vi "New JSON ([]).vi"(8 "error in (no error)":errorcluster) -> (0 "error out":errorcluster, 3 "JSON Value out":refnum<class "JSON Value.lvclass">)   [LabVIEW 2017, in "JSON Value.lvclass"]
doc: "Creates a new empty JSON Array"
uses:
  JSON Value.lvclass
  JSON Types.ctl
  JSON Value.lvclass/JSON Value.ctl
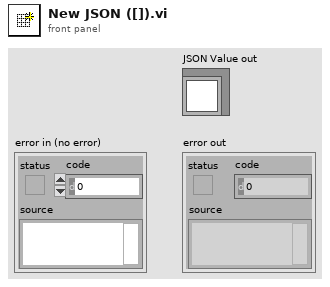
[diagram p1: front panel]
types:
  T1 = typedef "JSON Value.lvclass/JSON Types.ctl" = enum16{"String", "Numeric", "Boolean", "NULL", "Object", "Array"}
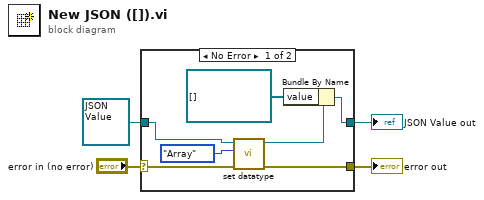
[diagram p0: block diagram]
diagram:
  n1 = case shown="No Error" "error in (no error)" {
    selector: "error in (no error)" -> [w11 w13]
    tunnel: [w10 w13] -> w3
    tunnel: [w6 w12] -> w2
    tunnel: refnum<class "JSON Value.lvclass"> refnum ("JSON out") -> [w9 w12]
    frame No Error {
      n2 = call "set datatype.vi"("error in (no error)"=w11, "datatype"=JSON_Types."Array", "JSON Helper in"=w9) -> ("error out"=w10:errorcluster, "JSON Helper out"=w7:refnum<class "JSON Value.lvclass">)  [unwired: 7 in]
      n3 = Bundle By Name(cluster=w7, "value"=refnum<class "JSON Value.lvclass">[] [] ("JSON out")) -> (w6:refnum<class "JSON Value.lvclass">)
    }
    frame Error {
    }
  }
  "error out" <- w3
  "JSON Value out" <- w2
